vi "TxtToExcelTimeTest.vi"() -> ()   [LabVIEW 2016]
panel:
  out "v3 Time":u32
  out "error out 2":errorcluster caption="error out"
  out "v4 Time":u32
  out "error out":errorcluster
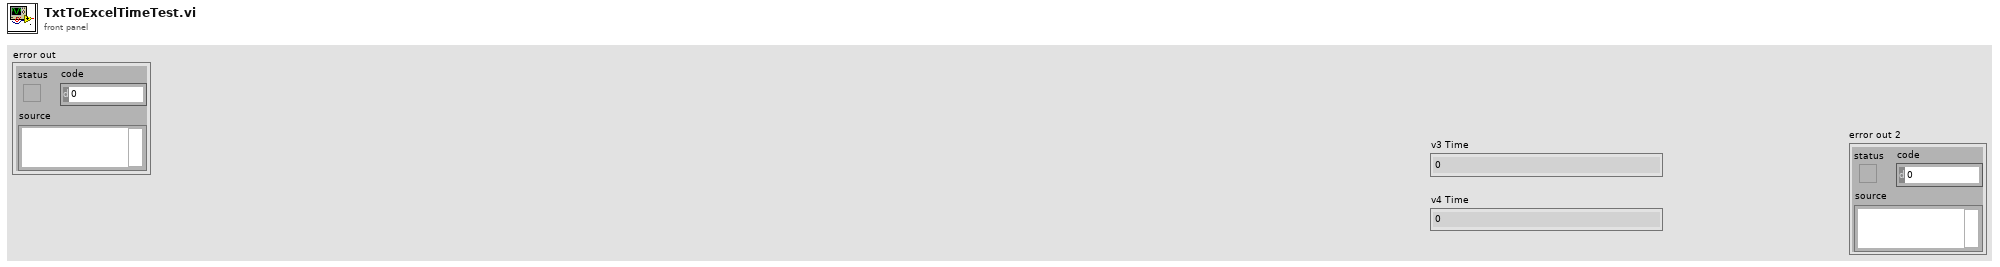
[diagram p1: front panel]
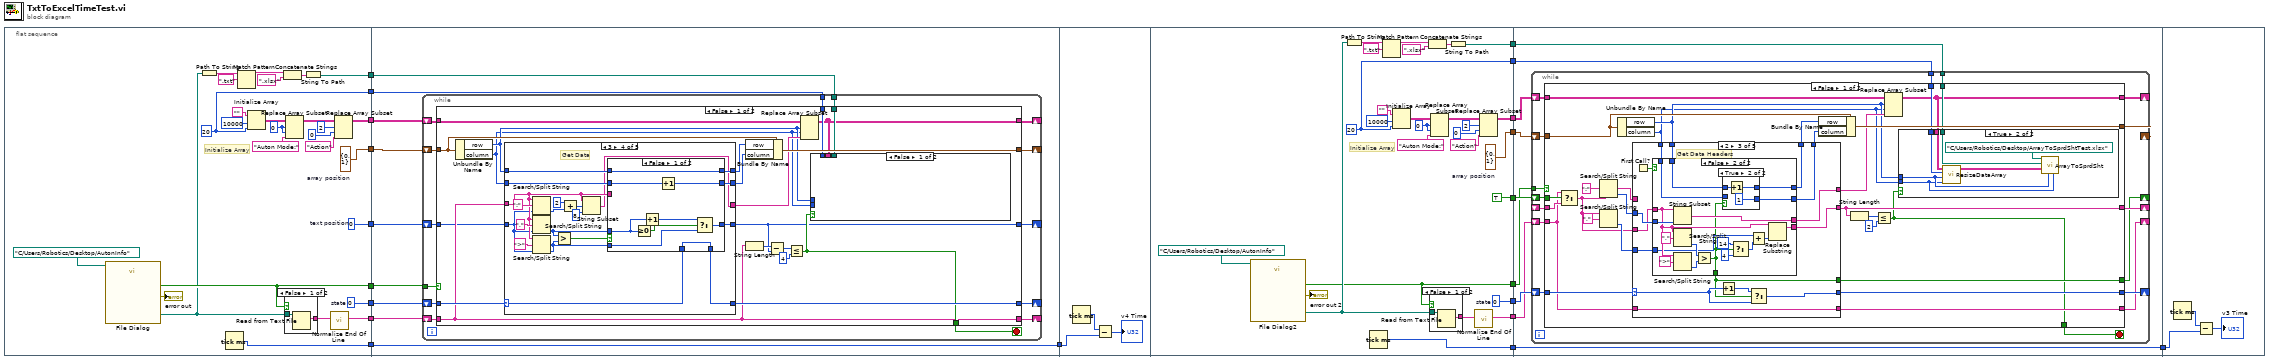
[diagram p0: block diagram]
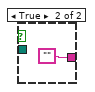
[diagram p2: hidden frame]
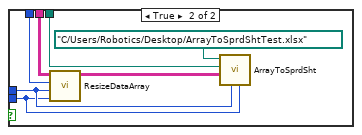
[diagram p3: hidden frame]
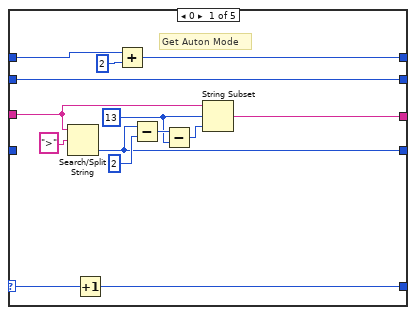
[diagram p4: hidden frame]
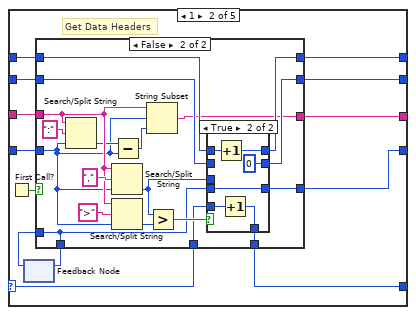
[diagram p5: hidden frame]
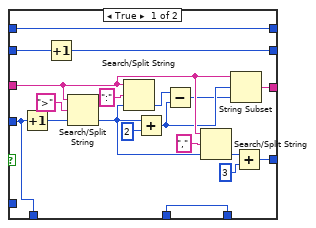
[diagram p6: hidden frame]
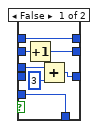
[diagram p7: hidden frame]
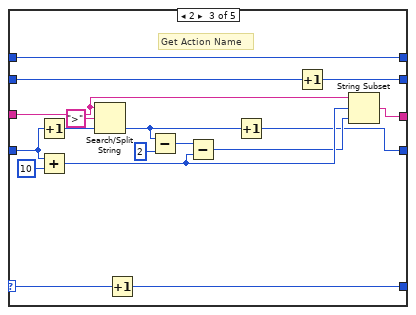
[diagram p8: hidden frame]
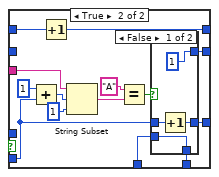
[diagram p9: hidden frame]
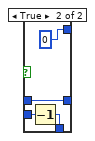
[diagram p10: hidden frame]
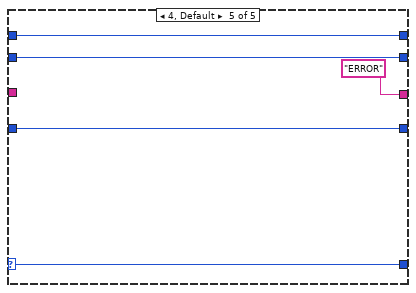
[diagram p11: hidden frame]
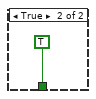
[diagram p12: hidden frame]
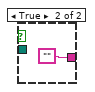
[diagram p13: hidden frame]
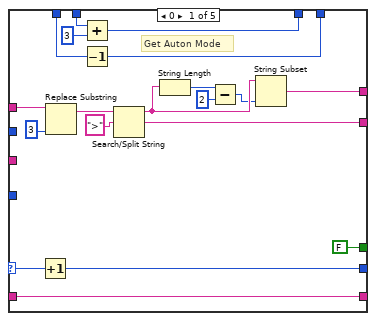
[diagram p15: hidden frame]
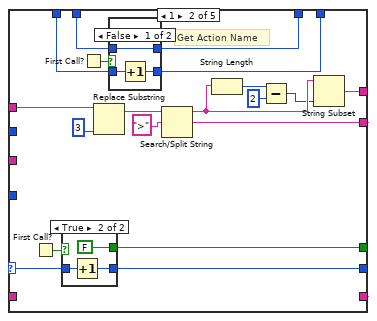
[diagram p16: hidden frame]
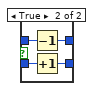
[diagram p17: hidden frame]
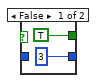
[diagram p18: hidden frame]
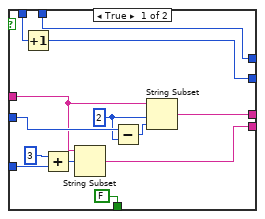
[diagram p19: hidden frame]
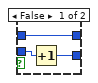
[diagram p20: hidden frame]
diagram:
  n1 = flat-sequence {
    tunnel: [w45] -> w20
    tunnel: [w44] -> w19
    tunnel: [w42] -> w18
    tunnel: [w39] -> w17
    tunnel: [w31] -> w16
    tunnel: [w26] -> w15
    tunnel: [w23] -> w14
    tunnel: [w22] -> w13
    tunnel: [w21] -> w11
    tunnel: w20 -> [w56]
    tunnel: w19 -> [w55]
    tunnel: w18 -> [w54]
    tunnel: w17 -> [w58]
    tunnel: w16 -> [w59]
    tunnel: w15 -> [w52]
    tunnel: w14 -> [w53]
    tunnel: w13 -> [w57]
    tunnel: [w51] -> w12
    tunnel: w11 -> [w51]
    tunnel: w12 -> [w254]
    tunnel: [w264] -> w10
    tunnel: [w263] -> w9
    tunnel: [w262] -> w8
    tunnel: [w261] -> w7
    tunnel: [w260] -> w6
    tunnel: [w259] -> w5
    tunnel: [w258] -> w4
    tunnel: [w257] -> w3
    tunnel: [TRUE] -> w2
    tunnel: w10 -> [w291]
    tunnel: w9 -> [w294]
    tunnel: w8 -> [w293]
    tunnel: w7 -> [w286]
    tunnel: w6 -> [w289]
    tunnel: w5 -> [w290]
    tunnel: w4 -> [w288]
    tunnel: w3 -> [w287]
    tunnel: w2 -> [w292]
    tunnel: [w286] -> w1
    tunnel: w1 -> [w492]
    frame #0 {
      w22 = 0  # text position
      w37 = 0 ("index (row)")
      w39 = cluster{"row":i32, "column":i32} {"row"=0, "column"=1}  # array position
      w23 = 20 ("Column Max")
      w44 = 0  # state
      # "Initialize Array"
      n2 = call "File Dialog"("start path"=path "C:/Users/Robotics/Desktop/AutonInfo") -> ("selected path"=w30:path, "cancelled"=w45:bool, "error out"=→"error out":errorcluster)  [unwired: 11 in, 1 out]
      n3 = Path To String(path=w30) -> (string=w29:string)
      n4 = Tick Count (ms)() -> (millisecond timer value=w21:u32)
      n5 = Match Pattern(string=w29, regular expression=".txt") -> (before substring=w25:string)  [unwired: 1 in, 3 out]
      n6 = Initialize Array("", 10000 ("Row Max"), w23) -> (w38:string[][])
      n7 = Concatenate Strings(w25, ".xlsx" ("string")) -> (w27:string)
      n8 = case shown="False" w45 {
        tunnel: w30 -> [w49 _]
        tunnel: [w48 ""] -> w43
        frame False {
          n9 = Read from Text File(file (use dialog)=w49) -> (text=w48:string)  [unwired: 3 in, 3 out]
        }
        frame True {
        }
      }
      n10 = Replace Array Subset(array=w38, new element="Auton Mode:" ("new element/subarray"), index (row)=w37, index (col)=w37) -> (w35:string[][])
      n11 = String To Path(string=w27) -> (path=w26:path)
      n12 = call <vilib>:"Normalize End Of Line.vi"("string in"=w43) -> ("string out"=w42:string)  [unwired: 7 in]
      n13 = Replace Array Subset(array=w35, new element="Action" ("new element/subarray"), index (row)=2, index (col)=0 ("disabled index (col)")) -> (w31:string[][])
    }
    frame #1 {
      n14 = while {
        tunnel: w56 -> [w73]
        shift-right: [w70] -> _
        shift-left: w55 -> [w71]
        shift-right: [w69] -> _
        shift-left: w54 -> [w68]
        shift-right: [w64] -> _
        shift-left: w59 -> [w66]
        shift-right: [w65] -> _
        shift-left: w58 -> [w67]
        tunnel: w52 -> [w63]
        tunnel: w53 -> [w62]
        shift-right: [w61] -> _
        shift-left: w57 -> [w60]
        stop <- w72 stop-if-true
        n15 = case shown="False" w73 {
          tunnel: [w84 TRUE] -> w72
          tunnel: w71 -> [w93 _]
          tunnel: [w92 _] -> w70
          tunnel: [w78 _] -> w69
          tunnel: w68 -> [w78 _]
          tunnel: w67 -> [w89 _]
          tunnel: w66 -> [w88 _]
          tunnel: [w90 _] -> w65
          tunnel: [w79 _] -> w64
          tunnel: w63 -> [w83 _]
          tunnel: w62 -> [w80 _]
          tunnel: [w76 _] -> w61
          tunnel: w60 -> [w74 _]
          frame False {
            n16 = Unbundle By Name(w89) -> ("row"=w82:i32, "column"=w81:i32)
            n17 = case shown="3" w93 {
              selector: w93 -> [w110 w116 w190 w204 w251]
              tunnel: [w113 w127 w195 w198 "ERROR" ("string out")] -> w87
              tunnel: w82 -> [w112 w126 w193 w210 w250]
              tunnel: [w108 w123 w193 w209 w250] -> w86
              tunnel: w81 -> [w101 w125 w194 w213 w249]
              tunnel: [w101 w122 w192 w212 w249] -> w85
              tunnel: [w109 w115 w191 w203 w251] -> w92
              tunnel: w78 -> [w106 w121 w184 w202 _]
              tunnel: [w102 w117 w179 w205 w248] -> w76
              tunnel: w74 -> [_ w119 w186 w201 w248]
              frame 0 {
                w104 = 13 ("y")
                # "Get Auton Mode"
                n18 = Search/Split String(string=w106, search string/char (-)=">") -> (offset of match=w102:i32)  [unwired: 1 in, 2 out]
                n19 = Increment(x=w110) -> (x+1=w109:i32)
                n20 = Add(x=w112, y=2) -> (x+y=w108:i32)
                n21 = Subtract(x=w102, y=2) -> (x-y=w105:i32)
                n22 = Subtract(x=w105, y=w104) -> (x-y=w103:i32)
                n23 = String Subset(string=w106, offset (0)=w104, length (rest)=w103) -> (substring=w113:string)
              }
              frame 1 {
                # "Get Data Headers"
                n24 = First Call?() -> (First Call?: T/F=w124:bool)
                n25 = feedback #1() -> (w118:i32)  [unwired: 1 in]
                n26 = case shown="False" w124 {
                  tunnel: [w146 w148] -> w127
                  tunnel: w126 -> [w143 w160]
                  tunnel: [w143 w159] -> w123
                  tunnel: w125 -> [w145 w165]
                  tunnel: [w144 w164] -> w122
                  tunnel: w121 -> [w139 w157]
                  tunnel: [w138 w152] -> w120
                  tunnel: w119 -> [w138 w154]
                  tunnel: w118 -> [_ w152]
                  tunnel: [w129 w149] -> w117
                  tunnel: w116 -> [w128 w151]
                  tunnel: [w128 w150] -> w115
                  frame True {
                    n27 = Increment(x=w138) -> (x+1=w137:i32)
                    n28 = Increment(x=w145) -> (x+1=w144:i32)
                    n29 = Search/Split String(string=w139, search string/char (-)=">", offset (0)=w137) -> (offset of match=w136:i32)  [unwired: 2 out]
                    n30 = Search/Split String(string=w139, search string/char (-)=":", offset (0)=w136) -> (offset of match=w134:i32)  [unwired: 2 out]
                    n31 = Add(x=w136, y=2 ("offset of match")) -> (x+y=w133:i32)
                    n32 = Subtract(x=w134, y=w133) -> (x-y=w132:i32)
                    n33 = Search/Split String(string=w139, search string/char (-)=",", offset (0)=w136) -> (offset of match=w130:i32)  [unwired: 2 out]
                    n34 = String Subset(string=w139, offset (0)=w133, length (rest)=w132) -> (substring=w146:string)
                    n35 = Add(x=w130, y=3 ("offset of match")) -> (x+y=w129:i32)
                  }
                  frame False {
                    n36 = Search/Split String(string=w157, search string/char (-)=":", offset (0)=w154) -> (offset of match=w156:i32)  [unwired: 2 out]
                    n37 = Search/Split String(string=w157, search string/char (-)=",", offset (0)=w154) -> (offset of match=w147:i32)  [unwired: 2 out]
                    n38 = Search/Split String(string=w157, search string/char (-)=">", offset (0)=w154) -> (offset of match=w161:i32)  [unwired: 2 out]
                    n39 = Subtract(x=w156, y=w154) -> (x-y=w155:i32)
                    n40 = String Subset(string=w157, offset (0)=w154, length (rest)=w155) -> (substring=w148:string)
                    n41 = Greater?(x=w147, y=w161) -> (0:w153:bool)
                    n42 = case shown="True" w153 {
                      tunnel: w165 -> [w172 _]
                      tunnel: [w171 0] -> w164
                      tunnel: w160 -> [w170 w177]
                      tunnel: [w170 w176] -> w159
                      tunnel: w152 -> [_ w175]
                      tunnel: [w169 w175] -> w149
                      tunnel: w151 -> [w168 w174]
                      tunnel: [w168 w173] -> w150
                      tunnel: w147 -> [w167 _]
                      frame False {
                        n43 = Increment(x=w172) -> (x+1=w171:i32)
                        n44 = Add(x=w167, y=3 ("x")) -> (x+y=w169:i32)
                      }
                      frame True {
                        n45 = Increment(x=w177) -> (x+1=w176:i32)
                        n46 = Increment(x=w174) -> (x+1=w173:i32)
                      }
                    }
                  }
                }
                n47 = feedback-in #1(w120) -> ()
              }
              frame 2 {
                # "Get Action Name"
                n48 = Increment(x=w186) -> (x+1=w188:i32)
                n49 = Add(x=w186, y=10) -> (x+y=w182:i32)
                n50 = Search/Split String(string=w184, search string/char (-)=">", offset (0)=w188) -> (offset of match=w180:i32)  [unwired: 2 out]
                n51 = Increment(x=w190) -> (x+1=w191:i32)
                n52 = Subtract(x=w180, y=2) -> (x-y=w183:i32)
                n53 = Subtract(x=w183, y=w182) -> (x-y=w181:i32)
                n54 = Increment(x=w180) -> (x+1=w179:i32)
                n55 = Increment(x=w194) -> (x+1=w192:i32)
                n56 = String Subset(string=w184, offset (0)=w182, length (rest)=w181) -> (substring=w195:string)
              }
              frame 3 {
                # "Get Data"
                n57 = Search/Split String(string=w202, search string/char (-)=":", offset (0)=w201) -> (offset of match=w207:i32)  [unwired: 2 out]
                n58 = Search/Split String(string=w202, search string/char (-)=",", offset (0)=w201) -> (offset of match=w196:i32)  [unwired: 2 out]
                n59 = Search/Split String(string=w202, search string/char (-)=">", offset (0)=w201) -> (offset of match=w197:i32)  [unwired: 2 out]
                n60 = Greater?(x=w196, y=w197) -> (0:w211:bool)
                n61 = Add(x=2 ("y"), y=w207) -> (x+y=w200:i32)
                n62 = String Subset(string=w202, offset (0)=w200, length (rest)=8 ("y")) -> (substring=w198:string)
                n63 = case shown="False" w211 {
                  tunnel: w213 -> [w224 _]
                  tunnel: [w223 w229] -> w212
                  tunnel: w210 -> [w222 w236]
                  tunnel: [w222 w235] -> w209
                  tunnel: w196 -> [w217 _]
                  tunnel: [w220 w225] -> w205
                  tunnel: w204 -> [w221 w228]
                  tunnel: [w221 w227] -> w203
                  tunnel: w202 -> [_ w233]
                  tunnel: w197 -> [w216 w226]
                  frame False {
                    n64 = Greater Or Equal To 0?(x=w217) -> (x >= 0?=w219:bool)
                    n65 = Increment(x=w217) -> (x+1=w218:i32)
                    n66 = Increment(x=w224) -> (x+1=w223:i32)
                    n67 = Select(t=w218, s=w219, f=w216) -> (s? t:f=w220:i32)
                  }
                  frame True {
                    n68 = Add(x=1 ("y"), y=w226) -> (x+y=w231:i32)
                    n69 = Increment(x=w236) -> (x+1=w235:i32)
                    n70 = String Subset(string=w233, offset (0)=w231, length (rest)=1 ("length (rest)")) -> (substring=w238:string)
                    n71 = Equal?(x="A", y=w238) -> (x = y?=w230:bool)
                    n72 = case shown="False" w230 {
                      tunnel: [1 ("length (rest)") 0 ("length (rest)")] -> w229
                      tunnel: w228 -> [w239 w245]
                      tunnel: [w239 w244] -> w227
                      tunnel: w226 -> [w242 w243]
                      tunnel: [w241 w243] -> w225
                      frame False {
                        n73 = Increment(x=w242) -> (x+1=w241:i32)
                      }
                      frame True {
                        n74 = Decrement(x=w245) -> (x-1=w244:i32)
                      }
                    }
                  }
                }
              }
              frame 4, Default {
              }
            }
            n75 = Bundle By Name(cluster=w89, "row"=w86, "column"=w85) -> (w90:cluster{"row":i32, "column":i32})
            n76 = String Length(string=w78) -> (length=w77:i32)
            n77 = Subtract(x=w77, y=w76) -> (x-y=w75:i32)
            n78 = Less Or Equal?(x=w75, y=4) -> (x <= y?=w84:bool)
            n79 = Replace Array Subset(array=w88, new element=w87, index (row)=w82, index (col)=w81) -> (w79:string[][])
            n80 = case shown="False" w84 {
              tunnel: w79 -> [_ w98]
              tunnel: w83 -> [_ w99]
              tunnel: w82 -> [_ w95]
              tunnel: w81 -> [_ w94]
              tunnel: w80 -> [_ w97]
              frame False {
              }
              frame True {
                n81 = call "ResizeDataArray.vi"("Column"=w94, "Row"=w95, "Column Max"=w97, "Input Array"=w98) -> ("Output Array"=w96:string[][])  [unwired: 3 in]
                n82 = call "ArrayToSprdSht.vi"("Column End"=w94, "Row End"=w95, "TextArray"=w96, "report file path"=w99, "template (empty)"=path "C:/Users/Robotics/Desktop/ArrayToSprdShtTest.xlsx" ("file path (dialog if empty)")) -> ()  [unwired: 7 in]
              }
            }
          }
          frame True {
          }
        }
      }
    }
    frame #2 {
      n83 = Tick Count (ms)() -> (millisecond timer value=w255:u32)
      n84 = Subtract(x=w255, y=w254) -> (x-y=→"v4 Time":u32)
    }
    frame #3 {
      w276 = 0 ("index (row)")
      w259 = cluster{"row":i32, "column":i32} {"row"=0, "column"=1}  # array position
      w258 = 20 ("Column Max")
      w263 = 0  # state
      # "Initialize Array"
      n85 = call "File Dialog2"("start path"=path "C:/Users/Robotics/Desktop/AutonInfo") -> ("selected path"=w270:path, "cancelled"=w264:bool, "error out"=→"error out 2":errorcluster)  [unwired: 11 in, 1 out]
      n86 = Path To String(path=w270) -> (string=w269:string)
      n87 = Tick Count (ms)() -> (millisecond timer value=w261:u32)
      n88 = Match Pattern(string=w269, regular expression=".txt") -> (before substring=w266:string)  [unwired: 1 in, 3 out]
      n89 = Initialize Array("", 10000 ("Row Max"), w258) -> (w277:string[][])
      n90 = Concatenate Strings(w266, ".xlsx" ("string")) -> (w267:string)
      n91 = case shown="False" w264 {
        tunnel: w270 -> [w284 _]
        tunnel: [w283 ""] -> w280
        frame False {
          n92 = Read from Text File(file (use dialog)=w284) -> (text=w283:string)  [unwired: 3 in, 3 out]
        }
        frame True {
        }
      }
      n93 = Replace Array Subset(array=w277, new element="Auton Mode:" ("new element/subarray"), index (row)=w276, index (col)=w276) -> (w274:string[][])
      n94 = String To Path(string=w267) -> (path=w257:path)
      n95 = call <vilib>:"Normalize End Of Line.vi"("string in"=w280) -> ("string out"=w262:string)  [unwired: 7 in]
      n96 = Replace Array Subset(array=w274, new element="Action" ("new element/subarray"), index (row)=2, index (col)=0 ("disabled index (col)")) -> (w260:string[][])
    }
    frame #4 {
      n97 = while {
        tunnel: w291 -> [w310]
        shift-right: [w307] -> _
        shift-left: _ -> [w309]
        shift-right: [w305] -> _
        shift-left: w294 -> [w306]
        shift-right: [w303] -> _
        shift-left: w292 -> [w304]
        shift-right: [w302] -> _
        shift-left: w293 -> [w301]
        shift-right: [w297] -> _
        shift-left: w289 -> [w299]
        shift-right: [w298] -> _
        shift-left: w290 -> [w300]
        tunnel: w287 -> [w296]
        tunnel: w288 -> [w295]
        stop <- w308 stop-if-true
        n98 = case shown="False" w310 {
          tunnel: w309 -> [w331 _]
          tunnel: [w316 TRUE] -> w308
          tunnel: [w327 _] -> w307
          tunnel: w306 -> [w335 _]
          tunnel: [w334 _] -> w305
          tunnel: w304 -> [w329 _]
          tunnel: [w328 _] -> w303
          tunnel: [w324 _] -> w302
          tunnel: w301 -> [w323 _]
          tunnel: w300 -> [w321 _]
          tunnel: w299 -> [w320 _]
          tunnel: [w322 _] -> w298
          tunnel: [w311 _] -> w297
          tunnel: w296 -> [w315 _]
          tunnel: w295 -> [w312 _]
          frame False {
            n99 = Select(t=w323, s=w329, f=w331) -> (s? t:f=w330:string)
            n100 = Search/Split String(string=w330, search string/char (-)=":") -> (match + rest of string=w336:string, offset of match=w333:i32)  [unwired: 1 in, 1 out]
            n101 = Search/Split String(string=w330, search string/char (-)=",") -> (offset of match=w332:i32)  [unwired: 1 in, 2 out]
            n102 = Unbundle By Name(w321) -> ("row"=w314:i32, "column"=w313:i32)
            n103 = case shown="2" w335 {
              selector: w335 -> [w356 w371 w403 _ w490]
              tunnel: w336 -> [w346 w379 _ w448 _]
              tunnel: [w359 w378 w408 w453 _] -> w319
              tunnel: [w362 w375 w406 w454 _] -> w327
              tunnel: w314 -> [w358 w376 w405 w461 w488]
              tunnel: [w351 w374 w398 w460 w488] -> w318
              tunnel: w313 -> [w354 w377 w404 w464 w487]
              tunnel: [w350 w373 w397 w463 w487] -> w317
              tunnel: [w355 w372 w409 w457 w490] -> w334
              tunnel: w333 -> [_ _ w401 w471 _]
              tunnel: w332 -> [_ _ w407 _ _]
              tunnel: w330 -> [_ _ w396 w451 _]
              tunnel: [FALSE w369 w400 _ _] -> w328
              tunnel: [w352 w375 w399 w456 w489] -> w324
              tunnel: w323 -> [w352 _ w399 w456 w489]
              frame 0 {
                # "Get Auton Mode"
                n104 = Increment(x=w356) -> (x+1=w355:i32)
                n105 = Replace Substring(2:3 ("length (len. of substring)"), 5:w346) -> (1:w363:string)  [unwired: 2 in, 1 out]
                n106 = Add(x=w358, y=3) -> (x+y=w351:i32)
                n107 = Decrement(x=w354) -> (x-1=w350:i32)
                n108 = Search/Split String(string=w363, search string/char (-)=">") -> (substring before match=w360:string, match + rest of string=w362:string)  [unwired: 1 in, 1 out]
                n109 = String Length(string=w360) -> (length=w349:i32)
                n110 = Subtract(x=w349, y=2) -> (x-y=w348:i32)
                n111 = String Subset(string=w360, length (rest)=w348) -> (substring=w359:string)  [unwired: 1 in]
              }
              frame 1 {
                # "Get Action Name"
                n112 = First Call?() -> (First Call?: T/F=w370:bool)
                n113 = case shown="True" w370 {
                  tunnel: [3 ("f") w395] -> w372
                  tunnel: w371 -> [_ w394]
                  tunnel: [TRUE FALSE] -> w369
                  frame False {
                  }
                  frame True {
                    n114 = Increment(x=w394) -> (x+1=w395:i32)
                  }
                }
                n115 = First Call?() -> (First Call?: T/F=w368:bool)
                n116 = Replace Substring(2:3 ("length (len. of substring)"), 5:w379) -> (1:w382:string)  [unwired: 2 in, 1 out]
                n117 = case shown="False" w368 {
                  tunnel: w377 -> [w386 w390]
                  tunnel: w376 -> [w384 w389]
                  tunnel: [w384 w388] -> w374
                  tunnel: [w385 w387] -> w373
                  frame False {
                    n118 = Increment(x=w386) -> (x+1=w385:i32)
                  }
                  frame True {
                    n119 = Decrement(x=w389) -> (x-1=w388:i32)
                    n120 = Increment(x=w390) -> (x+1=w387:i32)
                  }
                }
                n121 = Search/Split String(string=w382, search string/char (-)=">") -> (substring before match=w380:string, match + rest of string=w375:string)  [unwired: 1 in, 1 out]
                n122 = String Length(string=w380) -> (length=w365:i32)
                n123 = Subtract(x=w365, y=2) -> (x-y=w366:i32)
                n124 = String Subset(string=w380, length (rest)=w366) -> (substring=w378:string)  [unwired: 1 in]
              }
              frame 2 {
                # "Get Data Headers"
                n125 = First Call?() -> (First Call?: T/F=w402:bool)
                n126 = case shown="False" w402 {
                  tunnel: w401 -> [w422 w437]
                  tunnel: [w421 w441] -> w408
                  tunnel: w407 -> [w419 w427]
                  tunnel: [w418 w436] -> w406
                  tunnel: [FALSE w426] -> w400
                  tunnel: w405 -> [w412 w425]
                  tunnel: [w412 w424] -> w398
                  tunnel: w404 -> [w414 w439]
                  tunnel: [w413 w438] -> w397
                  tunnel: w396 -> [w411 w435]
                  frame True {
                    w420 = 2 ("length (len. of substring)")
                    n127 = Increment(x=w414) -> (x+1=w413:i32)
                    n128 = Add(x=3, y=w419) -> (x+y=w415:i32)
                    n129 = String Subset(string=w411, offset (0)=w415) -> (substring=w418:string)  [unwired: 1 in]
                    n130 = Subtract(x=w422, y=w420) -> (x-y=w423:i32)
                    n131 = String Subset(string=w411, offset (0)=w420, length (rest)=w423) -> (substring=w421:string)
                  }
                  frame False {
                    n132 = String Subset(string=w435, length (rest)=w437) -> (substring=w441:string)  [unwired: 1 in]
                    n133 = Search/Split String(string=w435, search string/char (-)=",") -> (offset of match=w432:i32)  [unwired: 1 in, 2 out]
                    n134 = Search/Split String(string=w435, search string/char (-)=">") -> (offset of match=w431:i32)  [unwired: 1 in, 2 out]
                    n135 = Greater?(x=w432, y=w431) -> (0:w426:bool)
                    n136 = case shown="True" w426 {
                      tunnel: w439 -> [w444 _]
                      tunnel: [w443 1] -> w438
                      tunnel: w425 -> [w442 w446]
                      tunnel: [w442 w445] -> w424
                      frame False {
                        n137 = Increment(x=w444) -> (x+1=w443:i32)
                      }
                      frame True {
                        n138 = Increment(x=w446) -> (x+1=w445:i32)
                      }
                    }
                    n139 = Select(t=14, s=w426, f=4) -> (s? t:f=w428:i32)
                    n140 = Add(x=w427, y=w428) -> (x+y=w440:i32)
                    n141 = Replace Substring(2:w440, 5:w435) -> (1:w436:string)  [unwired: 2 in, 1 out]
                  }
                }
                n142 = Increment(x=w403) -> (x+1=w410:i32)
                n143 = Select(t=w410, s=w400, f=w403) -> (s? t:f=w409:i32)
              }
              frame 3 {
                # "Get Data"
                n144 = Add(x=w471, y=2) -> (x+y=w450:i32)
                n145 = String Subset(string=w451, offset (0)=w450, length (rest)=8 ("length (rest)")) -> (substring=w453:string)
                n146 = Search/Split String(string=w448, search string/char (-)=":", offset (0)=w450) -> (match + rest of string=w455:string, offset of match=w466:i32)  [unwired: 1 out]
                n147 = Search/Split String(string=w448, search string/char (-)=">") -> (match + rest of string=w449:string, offset of match=w465:i32)  [unwired: 1 in, 1 out]
                n148 = Greater?(x=w466, y=w465) -> (0:w462:bool)
                n149 = case shown="True" w462 {
                  tunnel: w464 -> [w476 _]
                  tunnel: [w475 w480] -> w463
                  tunnel: w461 -> [w474 w484]
                  tunnel: [w474 w483] -> w460
                  tunnel: [FALSE w479] -> w459
                  tunnel: w455 -> [w472 _]
                  tunnel: w449 -> [_ w478]
                  tunnel: [w472 w478] -> w454
                  frame False {
                    n150 = Increment(x=w476) -> (x+1=w475:i32)
                  }
                  frame True {
                    w477 = 1 ("length (rest)")
                    n151 = Increment(x=w484) -> (x+1=w483:i32)
                    n152 = String Subset(string=w478, offset (0)=w477, length (rest)=w477) -> (substring=w486:string)
                    n153 = Equal?(x="A", y=w486) -> (x = y?=w479:bool)
                    n154 = Select(t=0 ("length (rest)"), s=w479, f=1 ("length (rest)")) -> (s? t:f=w480:i32)
                  }
                }
                n155 = Select(t=1 ("length (rest)"), s=w459, f=3 ("length (rest)")) -> (s? t:f=w457:i32)
              }
              frame 4, Default {
              }
            }
            n156 = Bundle By Name(cluster=w321, "row"=w318, "column"=w317) -> (w322:cluster{"row":i32, "column":i32})
            n157 = String Length(string=w327) -> (length=w326:i32)
            n158 = Less Or Equal?(x=w326, y=2) -> (x <= y?=w316:bool)
            n159 = Replace Array Subset(array=w320, new element=w319, index (row)=w314, index (col)=w313) -> (w311:string[][])
            n160 = case shown="True" w316 {
              tunnel: w311 -> [_ w343]
              tunnel: w315 -> [_ w344]
              tunnel: w314 -> [_ w340]
              tunnel: w313 -> [_ w339]
              tunnel: w312 -> [_ w342]
              frame False {
              }
              frame True {
                n161 = call "ResizeDataArray.vi"("Column"=w339, "Row"=w340, "Column Max"=w342, "Input Array"=w343) -> ("Output Array"=w341:string[][])  [unwired: 3 in]
                n162 = call "ArrayToSprdSht.vi"("Column End"=w339, "Row End"=w340, "TextArray"=w341, "report file path"=w344, "template (empty)"=path "C:/Users/Robotics/Desktop/ArrayToSprdShtTest.xlsx" ("file path (dialog if empty)")) -> ()  [unwired: 7 in]
              }
            }
          }
          frame True {
          }
        }
      }
    }
    frame #5 {
      n163 = Tick Count (ms)() -> (millisecond timer value=w494:u32)
      n164 = Subtract(x=w494, y=w492) -> (x-y=→"v3 Time":u32)
    }
  }
